vi "_PC_Pub_Upd_Graph_Param.vi"(5 "TIC":refnum<vi>, 7 "Mass spectrum":refnum<vi>, 8 "error in (no error)":errorcluster, 10 "Init?(F)":bool, 11 "Ionisation":refnum<vi>) -> (0 "error out":errorcluster)   [LabVIEW 2018]
uses:
  <vilib>/Utility/miscctls.llb/LVMajorAndMinorColorsTypeDef.ctl
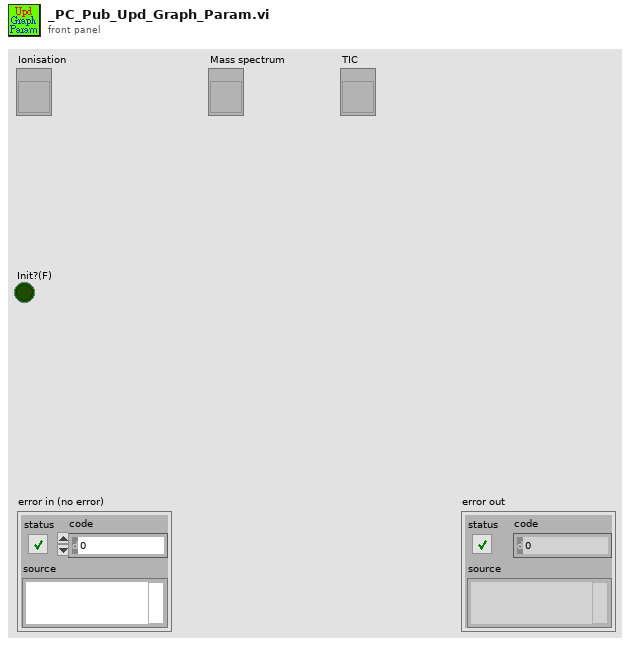
[diagram p1: front panel]
types:
  T1 = typedef "LVMajorAndMinorColorsTypeDef.ctl" = cluster{"Major Color":u32, "Minor Color":u32}
  T2 = cluster{"BGColor":u32, "GridX":bool, "GridY":bool, "LineColorArray":u32[], "LineWidthArray":u8[]}
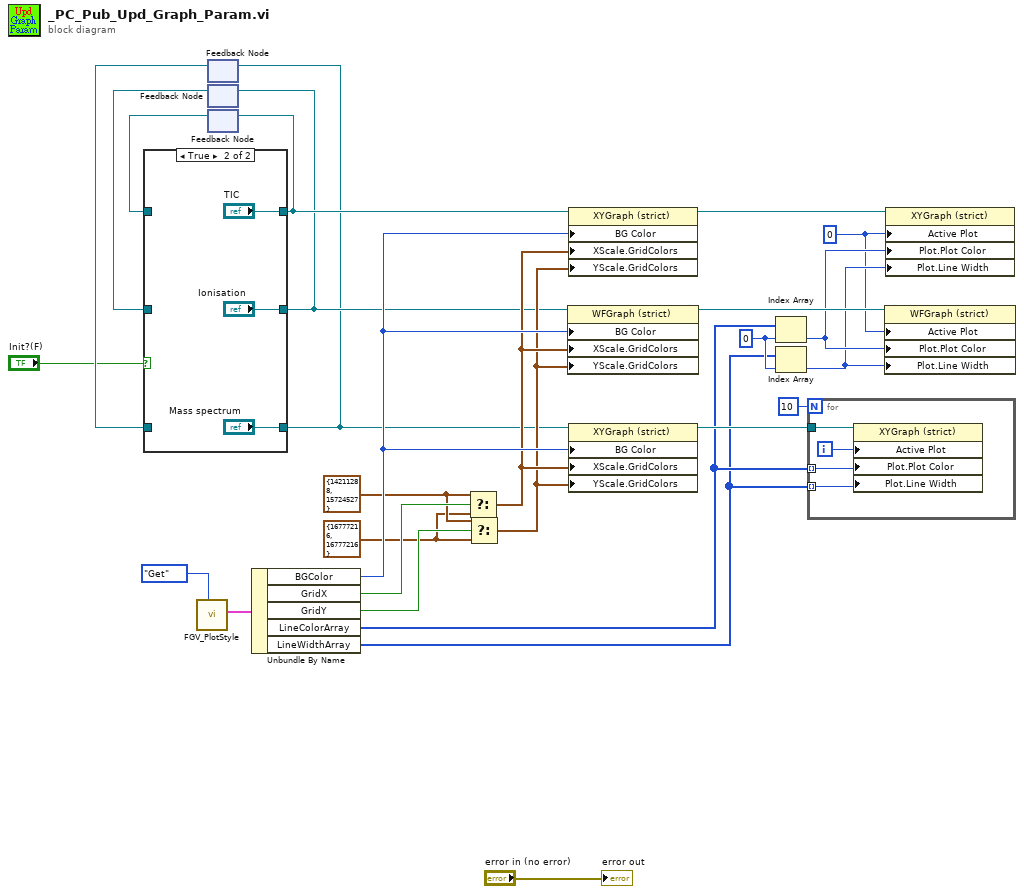
[diagram p0: block diagram]
diagram:
  w15 = 0 ("index")
  w12 = u32 0 ("Active Plot")
  w20 = T1 {"Major Color"=16777216, "Minor Color"=16777216} ("X Scale.Grid Colors")
  w21 = T1 {"Major Color"=14211288, "Minor Color"=15724527} ("X Scale.Grid Colors")
  n1 = call "FGV_PlotStyle.vi"("Function"=enum16{"Set", "Get"}."Get") -> ("Output Cluster"=w1:T2)  [unwired: 9 in, 1 out]
  n2 = feedback #1() -> (w6:refnum<vi>)  [unwired: 1 in]
  n3 = feedback #2() -> (w7:refnum<vi>)  [unwired: 1 in]
  n4 = feedback #3() -> (w9:refnum<vi>)  [unwired: 1 in]
  n5 = case shown="True" "Init?(F)" {
    tunnel: w9 -> [w30 _]
    tunnel: [w30 "TIC"] -> w8
    tunnel: w7 -> [w29 _]
    tunnel: w6 -> [w28 _]
    tunnel: [w29 "Ionisation"] -> w5
    tunnel: [w28 "Mass spectrum"] -> w4
    frame False {
    }
    frame True {
    }
  }
  n6 = feedback-in #1(w4) -> ()
  n7 = feedback-in #2(w5) -> ()
  n8 = feedback-in #3(w8) -> ()
  n9 = Unbundle By Name(w1) -> ("BGColor"=w27:u32, "GridX"=w26:bool, "GridY"=w25:bool, "LineColorArray"=w11:u32[], "LineWidthArray"=w10:u8[])
  n10 = Select(t=w21, s=w26, f=w20) -> (s? t:f=w23:T1)
  n11 = Select(t=w21, s=w25, f=w20) -> (s? t:f=w22:T1)
  n12 = property class="WFGraph (strict)"(reference=w5, "BG Color"=w27, "XScale.GridColors"=w23, "YScale.GridColors"=w22) -> (reference out=w18:refnum<vi>)  [unwired: 1 in, 1 out]
  n13 = property class="XYGraph (strict)"(reference=w8, "BG Color"=w27, "XScale.GridColors"=w23, "YScale.GridColors"=w22) -> (reference out=w19:refnum<vi>)  [unwired: 1 in, 1 out]
  n14 = property class="XYGraph (strict)"(reference=w4, "BG Color"=w27, "XScale.GridColors"=w23, "YScale.GridColors"=w22) -> (reference out=w17:refnum<vi>)  [unwired: 1 in, 1 out]
  n15 = Index Array(array=w11, index=w15) -> (element=w14:u32)
  n16 = Index Array(array=w10, index=w15) -> (element=w13:u8)
  n17 = for {
    N: 10 -> [_]
    tunnel: w17 -> [w37]
    tunnel: w11 -> [w35] mode=indexing
    tunnel: w10 -> [w34] mode=indexing
    i -> [w36]
    n18 = property class="XYGraph (strict)"(reference=w37, "Active Plot"=w36, "Plot.Plot Color"=w35, "Plot.Line Width"=w34) -> ()  [unwired: 1 in, 2 out]
  }
  n19 = property class="WFGraph (strict)"(reference=w18, "Active Plot"=w12, "Plot.Plot Color"=w14, "Plot.Line Width"=w13) -> ()  [unwired: 1 in, 2 out]
  n20 = property class="XYGraph (strict)"(reference=w19, "Active Plot"=w12, "Plot.Plot Color"=w14, "Plot.Line Width"=w13) -> ()  [unwired: 1 in, 2 out]
  "error out" <- "error in (no error)"
